vi "Combined Simulation SubVI for v6.0.vi"() -> (0 "Array":T3(array[cluster]), 1 "Cluster":T2)   [LabVIEW 2018]
panel:
  in  "Pressure Controls":T1 {"Line 5" scale=0.0..10.0; "Line 4" scale=0.0..10.0; "Line 3" scale=0.0..10.0; "Line 2" scale=0.0..10.0; "Line 1" scale=0.0..10.0}
  in  "Temperatures Control":T1 {"Line 5" scale=0.0..10.0; "Line 4" scale=0.0..10.0; "Line 3" scale=0.0..10.0; "Line 2" scale=0.0..10.0; "Line 1" scale=0.0..10.0}
  in  "Line Flowrate Control":T1 {"Line 5" scale=0.0..10.0; "Line 4" scale=0.0..10.0; "Line 3" scale=0.0..10.0; "Line 2" scale=0.0..10.0; "Line 1" scale=0.0..10.0}
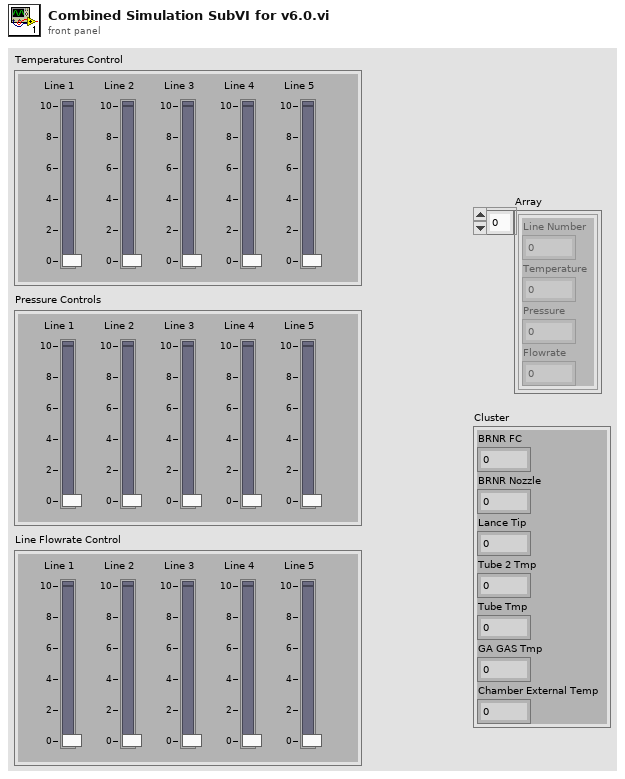
[diagram p1: front panel]
types:
  T1 = cluster{"Line 1":dbl, "Line 2":dbl, "Line 3":dbl, "Line 4":dbl, "Line 5":dbl}
  T2 = cluster{"BRNR FC":dbl, "BRNR Nozzle":dbl, "Lance Tip":dbl, "Tube 2 Tmp":dbl, "Tube Tmp":dbl, "GA GAS Tmp":dbl, "Chamber External Temp":dbl}
  T3 = cluster{"Line Number":dbl, "Temperature":dbl, "Pressure":dbl, "Flowrate":dbl}[]
  T4 = cluster{"Line Number":dbl, "Temperature":dbl, "Pressure":dbl, "Flowrate":dbl}
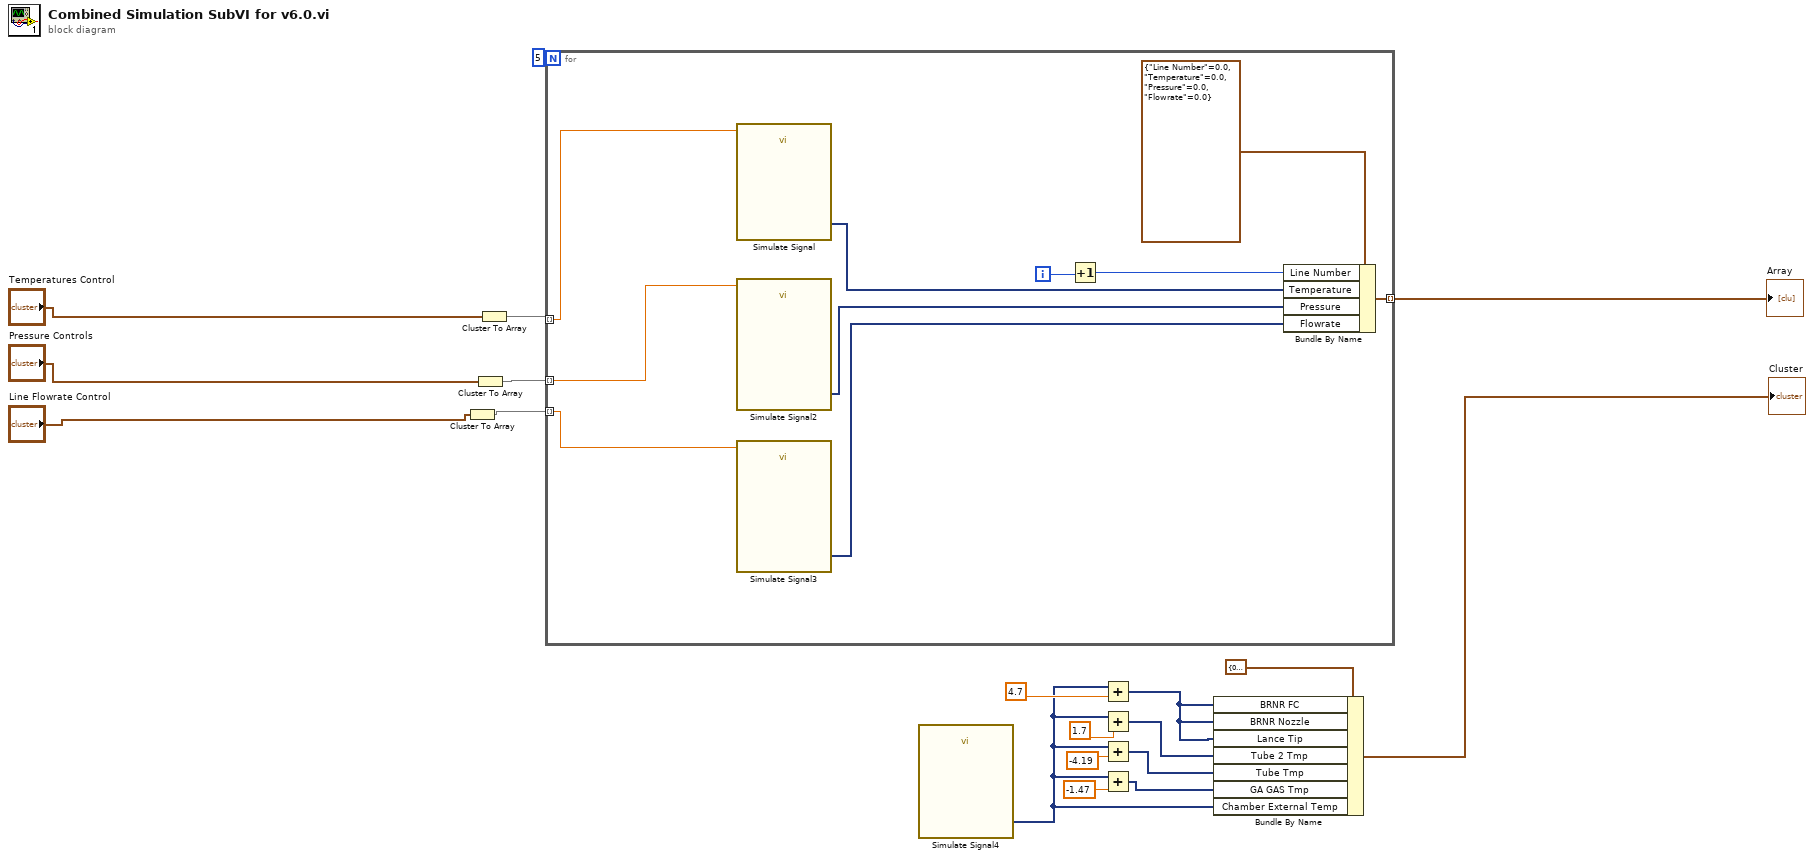
[diagram p0: block diagram]
diagram:
  n1 = Cluster To Array(cluster="Line Flowrate Control") -> (array=w4:dbl[])
  n2 = Cluster To Array(cluster="Pressure Controls") -> (array=w5:dbl[])
  n3 = Cluster To Array(cluster="Temperatures Control") -> (array=w6:dbl[])
  n4 = for {
    N: 5 -> [_]
    tunnel: [w29] -> w19 mode=indexing
    tunnel: w4 -> [w20] mode=indexing
    tunnel: w6 -> [w26] mode=indexing
    tunnel: w5 -> [w21] mode=indexing
    i -> [w27]
    n5 = call "Simulate Signal"("Offset"=w26) -> ("Temperature"=w25:dynamicdata)  [unwired: 13 in, 1 out]
    n6 = call "Simulate Signal2"("Offset"=w21) -> ("Pressure"=w23:dynamicdata)  [unwired: 13 in, 1 out]
    n7 = call "Simulate Signal3"("Offset"=w20) -> ("Flowrate"=w22:dynamicdata)  [unwired: 13 in, 1 out]
    n8 = Increment(x=w27) -> (x+1=w24:i32)
    n9 = Bundle By Name(cluster=T4 {"Line Number"=0.0, "Temperature"=0.0, "Pressure"=0.0, "Flowrate"=0.0}, "Line Number"=w24, "Temperature"=w25, "Pressure"=w23, "Flowrate"=w22) -> (w29:T4)
  }
  "Array" <- w19
  n10 = call "Simulate Signal4"() -> ("Rig Temperatures"=w8:dynamicdata)  [unwired: 14 in, 1 out]
  n11 = Add(x=w8, y=4.7) -> (x+y=w16:dynamicdata)
  n12 = Add(x=w8, y=1.7) -> (x+y=w14:dynamicdata)
  n13 = Add(x=w8, y=-4.19) -> (x+y=w12:dynamicdata)
  n14 = Add(x=w8, y=-1.47) -> (x+y=w10:dynamicdata)
  n15 = Bundle By Name(cluster=T2 {"BRNR FC"=0.0, "BRNR Nozzle"=0.0, "Lance Tip"=0.0, "Tube 2 Tmp"=0.0, "Tube Tmp"=0.0, "GA GAS Tmp"=0.0, "Chamber External Temp"=0.0}, "BRNR FC"=w16, "BRNR Nozzle"=w16, "Lance Tip"=w16, "Tube 2 Tmp"=w14, "Tube Tmp"=w12, "GA GAS Tmp"=w10, "Chamber External Temp"=w8) -> (→"Cluster":T2)
